vi "AO Create.vi"(8 "error in (no error)":errorcluster, 10 "Analog_Configuration_Parameters":T1, 11 "FC2901 in":refnum<class "FC2901.lvclass">) -> (0 "error out":errorcluster, 3 "FC2901 out":refnum<class "FC2901.lvclass">)   [LabVIEW 2021, in "FC2901.lvclass"]
uses:
  FC2901.lvclass
  FC2901.lvclass/FC2901.ctl
  <vilib>/NathanCo/Analog Tasks/Analog Output/Analog Output/Analog Output.lvclass
  <vilib>/NathanCo/Analog Tasks/Utilities/Analog Configuration Parameters.ctl
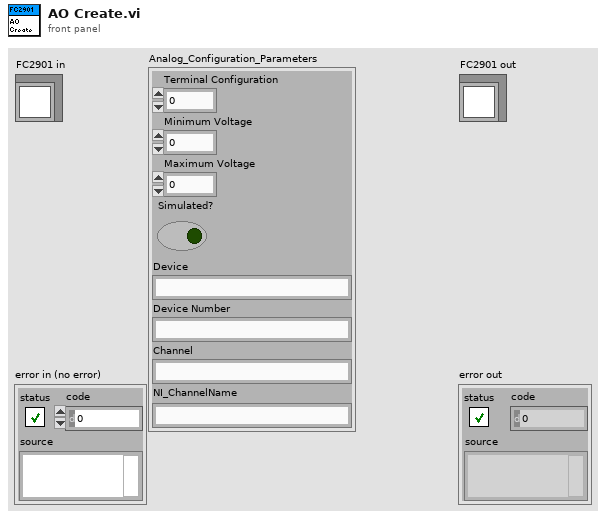
[diagram p1: front panel]
types:
  T1 = typedef "Analog Configuration Parameters.ctl" = cluster{"Terminal Configuration":i32, "Minimum Voltage":dbl, "Maximum Voltage":dbl, "Simulated?":bool, "Device":string, "Device Number":string, "Channel":string, "NI_ChannelName":string}
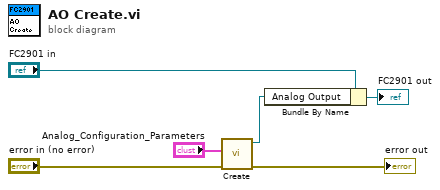
[diagram p0: block diagram]
diagram:
  n1 = call <vilib>:"Create.vi"("error in (no error)"="error in (no error)", "Analog_Configuration_Parameters"="Analog_Configuration_Parameters") -> ("error out"=→"error out":errorcluster, "Analog Output out"=w4:refnum<class "Analog Output.lvclass">)  [unwired: 8 in]
  n2 = Bundle By Name(cluster="FC2901 in", "Analog Output"=w4) -> (→"FC2901 out":refnum<class "FC2901.lvclass">)
